vi "Copy Class.vi"(5 "Parent Class Path":path, 7 "Template Path":path, 8 "error in (no error)":errorcluster, 9 "Class Name":string, 10 "Destination Directory":path, 11 "AppInst":refnum<vi>) -> (0 "error out":errorcluster, 2 "New Class Path":path)   [LabVIEW 2020, in "Message Maker.lvlib"]
uses:
  <resource>/Framework/Providers/MessageMakerProvider/_Message Maker/Message Maker.lvlib
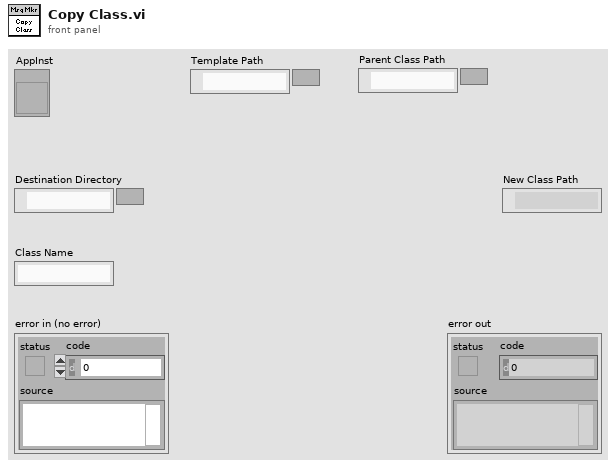
[diagram p1: front panel]
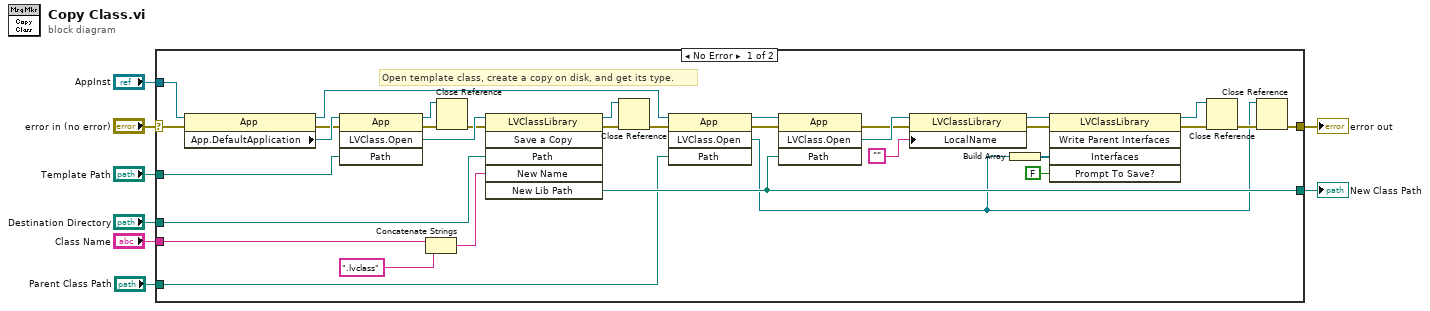
[diagram p0: block diagram]
diagram:
  n1 = case shown="No Error" "error in (no error)" {
    selector: "error in (no error)" -> [w34 w42]
    tunnel: "Template Path" -> [w33 _]
    tunnel: "Destination Directory" -> [w39 _]
    tunnel: [w30 _] -> w6
    tunnel: "Class Name" -> [w38 _]
    tunnel: [w21 w42] -> w4
    tunnel: "AppInst" -> [w18 _]
    tunnel: "Parent Class Path" -> [w16 _]
    frame No Error {
      # "Open template class, create a copy on disk, and get its type."
      n2 = property class="App"(reference=w18, error in=w34) -> (reference out=w17:refnum<vi>, error out=w31:errorcluster, "App.DefaultApplication"=w32:refnum<vi>)
      n3 = invoke class="App" method="LVClass.Open"(reference=w32, error in=w31, "Path"=w33) -> (reference out=w19:refnum<vi>, error out=w36:errorcluster, "LVClass.Open"=w41:refnum<vi>)  [unwired: 1 in, 1 out]
      n4 = Concatenate Strings(w38, ".lvclass" ("regular expression")) -> (w37:string)
      n5 = Close Reference(reference=w19, error in (no error)=w36) -> (error out=w20:errorcluster)
      n6 = invoke class="LVClassLibrary" method="Save a Copy"(reference=w41, error in=w20, "Path"=w39, "New Name"=w37) -> (reference out=w40:refnum<vi>, error out=w35:errorcluster, "New Lib Path"=w30:path)  [unwired: 2 in, 3 out]
      n7 = Close Reference(reference=w40, error in (no error)=w35) -> (error out=w28:errorcluster)
      n8 = invoke class="App" method="LVClass.Open"(reference=w17, error in=w28, "Path"=w16) -> (reference out=w26:refnum<vi>, error out=w27:errorcluster, "LVClass.Open"=w10:refnum<vi>)  [unwired: 1 in, 1 out]
      n9 = invoke class="App" method="LVClass.Open"(reference=w26, error in=w27, "Path"=w30) -> (error out=w25:errorcluster, "LVClass.Open"=w29:refnum<vi>)  [unwired: 1 in, 2 out]
      n10 = property class="LVClassLibrary"(reference=w29, error in=w25, "LocalName"="") -> (reference out=w13:refnum<vi>, error out=w24:errorcluster)
      n11 = Build Array(w10) -> (w9:refnum<vi>[])
      n12 = invoke class="LVClassLibrary" method="Write Parent Interfaces"(reference=w13, error in=w24, "Interfaces"=w9, "Prompt To Save?"=FALSE) -> (reference out=w12:refnum<vi>, error out=w14:errorcluster)  [unwired: 1 in, 3 out]
      n13 = Close Reference(reference=w12, error in (no error)=w14) -> (error out=w23:errorcluster)
      n14 = Close Reference(reference=w10, error in (no error)=w23) -> (error out=w21:errorcluster)
    }
    frame Error {
    }
  }
  "error out" <- w4
  "New Class Path" <- w6
